vi "Folder Creation.vi"(7 "Create New? (F)":bool, 11 "error in":errorcluster, 13 "Folder Name":T1) -> (4 "Tower Test File's - Folder Path":path, 8 "Selected Folder Path Out":path, 15 "error out":errorcluster)   [LabVIEW 2024]
uses:
  Host-Control's/DTT Test folder Name's.ctl
  9102cca0-df71-4fda-8ad0-13fbbf30117f.vi
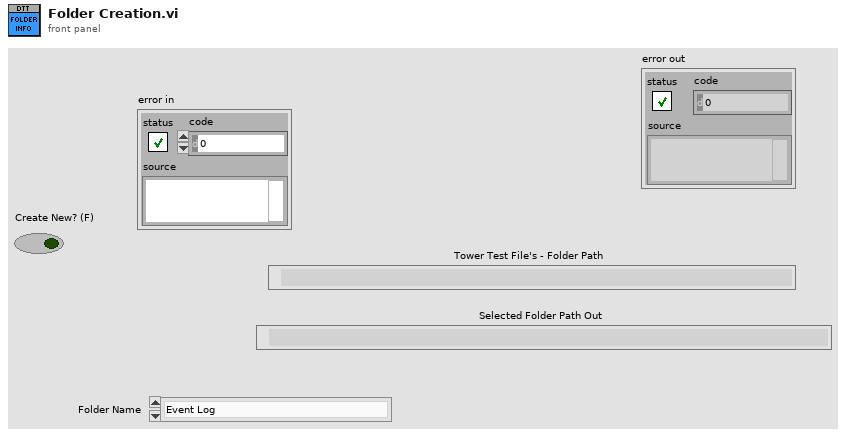
[diagram p1: front panel]
types:
  T1 = typedef "DTT Test folder Name's.ctl" = enum16{"Event Log", "Auto Sequence Configuration", "Channel Configuration's", "Test Data's"}
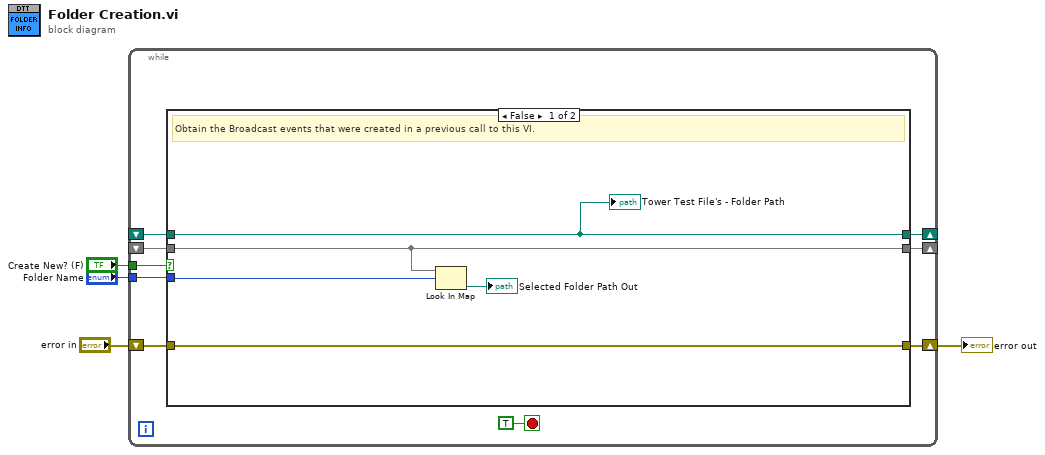
[diagram p0: block diagram]
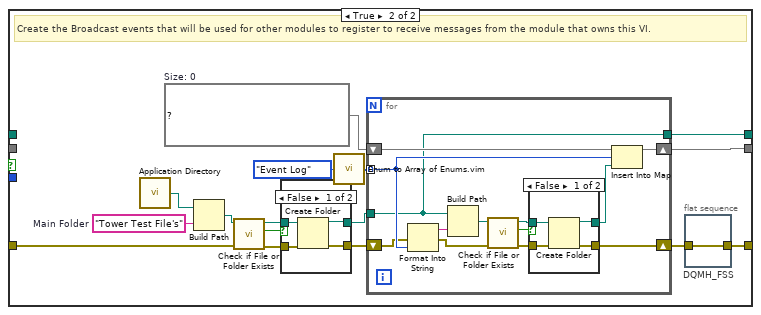
[diagram p2: hidden frame]
diagram:
  n1 = while {
    tunnel: "Create New? (F)" -> [w11]
    tunnel: "Folder Name" -> [w10]
    shift-right: [w9] -> w1
    shift-left: "error in" -> [w13]
    shift-right: [w12] -> _
    shift-left: _ -> [w8]
    shift-right: [w7] -> _
    shift-left: _ -> [w6]
    stop <- TRUE stop-if-true
    n2 = case shown="False" w11 {
      tunnel: w13 -> [w15 w23]
      tunnel: [w18 w25] -> w12
      tunnel: w8 -> [w18 _]
      tunnel: w10 -> [w16 _]
      tunnel: [w15 w20] -> w9
      tunnel: [w14 w19] -> w7
      tunnel: w6 -> [w14 _]
      frame False {
        # "Obtain the Broadcast events that were created in a previous call to this VI."
        n3 = Look In Map(map=w18, key=w16) -> (value=→"Selected Folder Path Out":path)  [unwired: 1 in, 1 out]
        "Tower Test File's - Folder Path" <- w14
      }
      frame True {
        w27 = "Tower Test File's"  # Main Folder
        w26 = map{T1, path} {}  # Size: 0
        # "Create the Broadcast events that will be used for other modules to register to receive messages from the module that owns this VI."
        n4 = call <vilib>:"Application Directory.vi"() -> ("Application Directory"=w28:path)
        n5 = Build Path(base path=w28, name or relative path=w27) -> (appended path=w29:path)
        n6 = call <vilib>:"Check if File or Folder Exists.vi"("error in (no error)"=w23, "path"=w29) -> ("error out"=w32:errorcluster, "file or folder exists?"=w30:bool, "dup path"=w31:path)  [unwired: 7 in]
        n7 = case shown="False" w30 {
          tunnel: w31 -> [w57 w59]
          tunnel: [w55 w59] -> w33
          tunnel: w32 -> [w56 w58]
          tunnel: [w54 w58] -> w34
          frame False {
            n8 = Create Folder(path (use dialog)=w57, error in=w56) -> (created path=w55:path, error out=w54:errorcluster)  [unwired: 1 in, 1 out]
          }
          frame True {
          }
        }
        n9 = call "Enum to Array of Enums.vim"("enum"=DTT_Test_folder_Name's."Event Log" ("Folder Name")) -> ("array of enums"=w21:T1[])
        n10 = for {
          tunnel: w33 -> [w35]
          shift-right: [w46] -> w24
          shift-left: w34 -> [w37]
          shift-right: [w41] -> w25
          shift-left: w26 -> [w42]
          tunnel: w21 -> [w38] mode=indexing
          tunnel: [w35] -> w19
          n11 = Format Into String(error in=w37, w38) -> (resulting string=w39:string, error out=w36:errorcluster)  [unwired: 2 in]
          n12 = Build Path(base path=w35, name or relative path=w39) -> (appended path=w47:path)
          n13 = call <vilib>:"Check if File or Folder Exists.vi"("error in (no error)"=w36, "path"=w47) -> ("error out"=w44:errorcluster, "file or folder exists?"=w45:bool, "dup path"=w43:path)  [unwired: 7 in]
          n14 = case shown="False" w45 {
            tunnel: w43 -> [w51 w53]
            tunnel: [w49 w53] -> w40
            tunnel: w44 -> [w50 w52]
            tunnel: [w48 w52] -> w46
            frame False {
              n15 = Create Folder(path (use dialog)=w51, error in=w50) -> (created path=w49:path, error out=w48:errorcluster)  [unwired: 1 in, 1 out]
            }
            frame True {
            }
          }
          n16 = Insert Into Map(map in=w42, key=w38, value=w40) -> (map out=w41:map{T1, path})  [unwired: 2 out]
        }
        n17 = flat-sequence "DQMH_FSS" {
          tunnel: [w60] -> w20
          tunnel: w24 -> [w60]
          frame #0 {
          }
        }
      }
    }
  }
  "error out" <- w1
